vi "Options Val error strings.vi"(5 "Array of error strings":string[](array[string])) -> (6 "Array of error strings out":string[](array[string]), 10 "Error":bool)   [LabVIEW 2011]
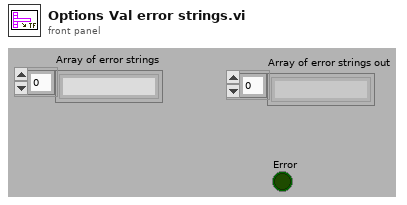
[diagram p1: front panel]
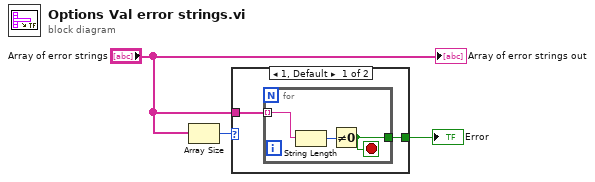
[diagram p0: block diagram]
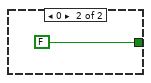
[diagram p2: hidden frame]
diagram:
  n1 = Array Size(array="Array of error strings") -> (size(s)=w3:i32)
  n2 = case shown="1, Default" w3 {
    tunnel: "Array of error strings" -> [w5 _]
    tunnel: [w4 FALSE] -> w2
    frame 1, Default {
      n3 = for {
        tunnel: w5 -> [w6] mode=indexing
        tunnel: [w7] -> w4
        stop <- w7 stop-if-true
        n4 = String Length(string=w6) -> (length=w8:i32)
        n5 = Not Equal To 0?(x=w8) -> (x != 0?=w7:bool)
      }
    }
    frame 0 {
    }
  }
  "Error" <- w2
  "Array of error strings out" <- "Array of error strings"
